vi "Build NT String Buffer.vi"(11 "String":string) -> (3 "Data Buffer":string)   [LabVIEW 2017]
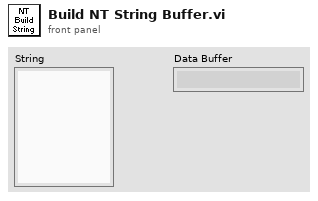
[diagram p1: front panel]
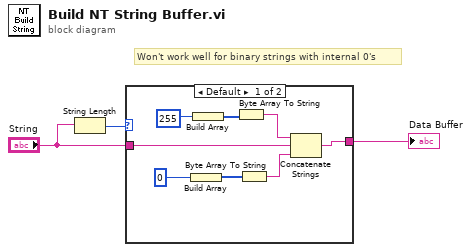
[diagram p0: block diagram]
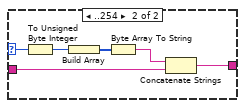
[diagram p2: hidden frame]
diagram:
  # "Won't work well for binary strings with internal 0's"
  n1 = String Length(string="String") -> (length=w3:i32)
  n2 = case shown="Default" w3 {
    selector: w3 -> [_ w17]
    tunnel: "String" -> [w9 w13]
    tunnel: [w8 w12] -> w1
    frame Default {
      n3 = Build Array(u8 0) -> (w4:u8[])
      n4 = Build Array(u8 255) -> (w7:u8[])
      n5 = Byte Array To String(unsigned byte array=w7) -> (string=w6:string)
      n6 = Byte Array To String(unsigned byte array=w4) -> (string=w5:string)
      n7 = Concatenate Strings(w6, w9, w5) -> (w8:string)
    }
    frame ..254 {
      n8 = To Unsigned Byte Integer(number=w17) -> (unsigned 8bit integer=w16:u8)
      n9 = Build Array(w16) -> (w15:u8[])
      n10 = Byte Array To String(unsigned byte array=w15) -> (string=w14:string)
      n11 = Concatenate Strings(w14, w13) -> (w12:string)
    }
  }
  "Data Buffer" <- w1
